vi "ExSub5strip.vi"(2 "error in (no error)":errorcluster, 3 "5 ROIS":T1, 4 "Camera Handle":u32) -> (0 "error out":errorcluster, 1 "Camera Handle":u32)   [LabVIEW 2010]
panel:
  # "ExSub5strip : this example programs up\n5 strips to collect."
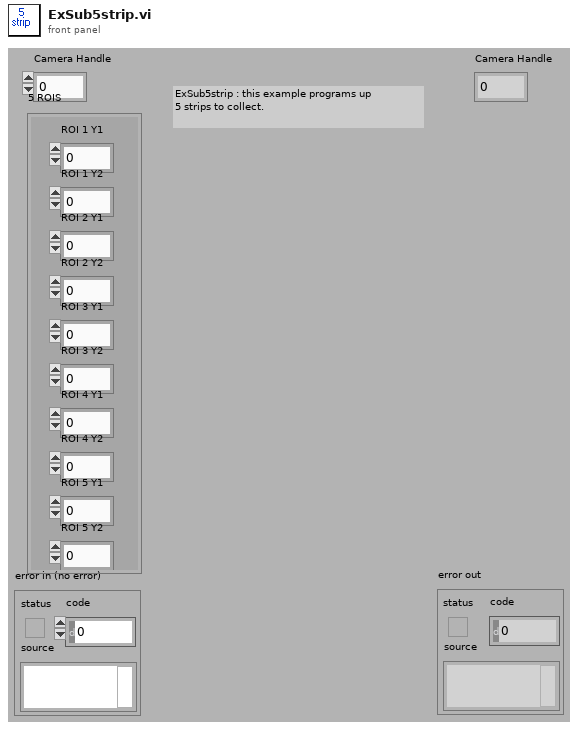
[diagram p1: front panel]
types:
  T1 = cluster{"ROI 1 Y1":u32, "ROI 1 Y2":u32, "ROI 2 Y1":u32, "ROI 2 Y2":u32, "ROI 3 Y1":u32, "ROI 3 Y2":u32, "ROI 4 Y1":u32, "ROI 4 Y2":u32, "ROI 5 Y1":u32, "ROI 5 Y2":u32}
  T2 = cluster{i32, "Xdim":u32, i32, "ROI 1 Y1":u32, "ROI 1 Y2":u32, u32}
  T3 = cluster{i32, "Xdim":u32, i32, "ROI 2 Y1":u32, "ROI 2 Y2":u32, u32}
  T4 = cluster{i32, "Xdim":u32, i32, "ROI 3 Y1":u32, "ROI 3 Y2":u32, u32}
  T5 = cluster{i32, "Xdim":u32, i32, "ROI 4 Y1":u32, "ROI 4 Y2":u32, u32}
  T6 = cluster{i32, "Xdim":u32, i32, "ROI 5 Y1":u32, "ROI 5 Y2":u32, u32}
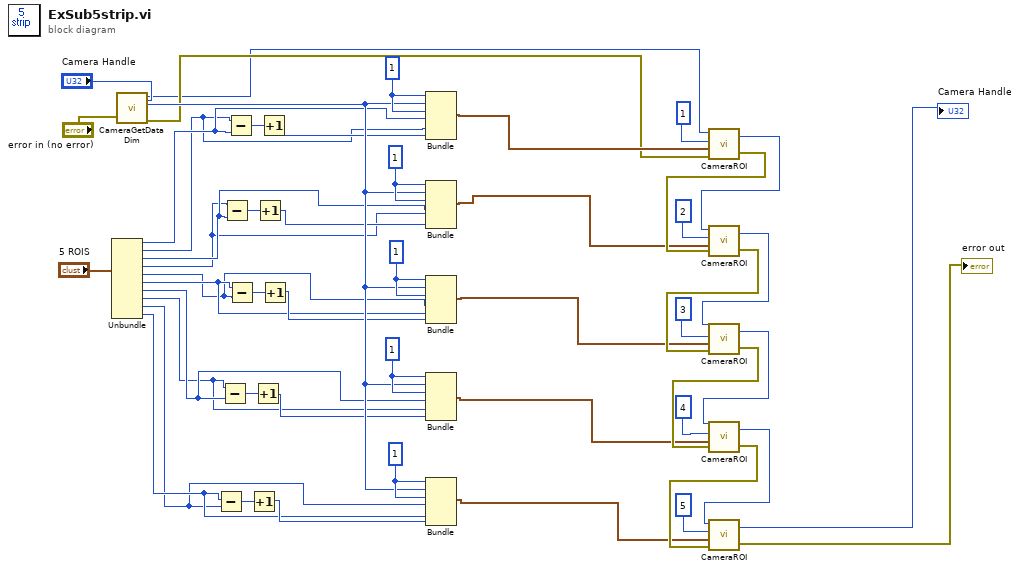
[diagram p0: block diagram]
diagram:
  w36 = 1
  w37 = 1
  w38 = 1
  w39 = 1
  w40 = 1
  n1 = Unbundle("5 ROIS") -> ("ROI 1 Y1"=w23:u32, "ROI 1 Y2"=w22:u32, "ROI 2 Y1"=w21:u32, "ROI 2 Y2"=w20:u32, "ROI 3 Y1"=w18:u32, "ROI 3 Y2"=w19:u32, "ROI 4 Y1"=w14:u32, "ROI 4 Y2"=w13:u32, "ROI 5 Y1"=w10:u32, "ROI 5 Y2"=w11:u32)
  n2 = call <userlib>:"CameraGetDataDim.vi"("Camera Handle"="Camera Handle", "error in"="error in (no error)") -> ("Camera Handle"=w7:u32, "Xdim"=w35:u32, "error out"=w8:errorcluster)  [unwired: 1 out]
  n3 = Subtract(x=w11, y=w10) -> (x-y=w28:u32)
  n4 = Subtract(x=w13, y=w14) -> (x-y=w29:u32)
  n5 = Subtract(x=w20, y=w21) -> (x-y=w31:u32)
  n6 = Subtract(x=w22, y=w23) -> (x-y=w33:u32)
  n7 = Subtract(x=w19, y=w18) -> (x-y=w30:u32)
  n8 = Increment(x=w28) -> (x+1=w24:u32)
  n9 = Increment(x=w29) -> (x+1=w25:u32)
  n10 = Increment(x=w31) -> (x+1=w27:u32)
  n11 = Increment(x=w33) -> (x+1=w32:u32)
  n12 = Increment(x=w30) -> (x+1=w26:u32)
  n13 = Bundle(w40, "Xdim"=w35, w40, "ROI 1 Y1"=w23, "ROI 1 Y2"=w22, w32) -> (w17:T2)  [unwired: 1 in]
  n14 = Bundle(w39, "Xdim"=w35, w39, "ROI 2 Y1"=w21, "ROI 2 Y2"=w20, w27) -> (w16:T3)  [unwired: 1 in]
  n15 = Bundle(w38, "Xdim"=w35, w38, "ROI 3 Y1"=w18, "ROI 3 Y2"=w19, w26) -> (w15:T4)  [unwired: 1 in]
  n16 = Bundle(w37, "Xdim"=w35, w37, "ROI 4 Y1"=w14, "ROI 4 Y2"=w13, w25) -> (w12:T5)  [unwired: 1 in]
  n17 = Bundle(w36, "Xdim"=w35, w36, "ROI 5 Y1"=w10, "ROI 5 Y2"=w11, w24) -> (w9:T6)  [unwired: 1 in]
  n18 = call <userlib>:"CameraROI.vi"("error in"=w8, "ROI Params"=w17, "ROI Index"=1, "Camera Handle"=w7) -> ("error out"=w44:errorcluster, "Camera Handle"=w6:u32)
  n19 = call <userlib>:"CameraROI.vi"("error in"=w44, "ROI Params"=w16, "ROI Index"=2, "Camera Handle"=w6) -> ("error out"=w43:errorcluster, "Camera Handle"=w5:u32)
  n20 = call <userlib>:"CameraROI.vi"("error in"=w43, "ROI Params"=w15, "ROI Index"=3, "Camera Handle"=w5) -> ("error out"=w42:errorcluster, "Camera Handle"=w4:u32)
  n21 = call <userlib>:"CameraROI.vi"("error in"=w42, "ROI Params"=w12, "ROI Index"=4, "Camera Handle"=w4) -> ("error out"=w41:errorcluster, "Camera Handle"=w3:u32)
  n22 = call <userlib>:"CameraROI.vi"("error in"=w41, "ROI Params"=w9, "ROI Index"=5, "Camera Handle"=w3) -> ("error out"=→"error out":errorcluster, "Camera Handle"=→"Camera Handle":u32)
